vi "Align to Ball.vi"   [LabVIEW 2013]
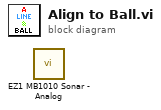
[diagram p0: block diagram]
diagram:
  n1 = call "EZ1 MB1010 Sonar - Analog.vi"() -> ()  [unwired: 1 in]
